vi "_Remote Set RF EN.vi"(4 "error in":errorcluster, 5 "RF EN (F)":bool, 6 "Q3? (F)":bool, 7 "Running (F)":bool) -> (0 "error out":errorcluster)   [LabVIEW 2012]
uses:
  Type/_RT Parameter.ctl
  Type/_RT Active Ch.ctl
  Type/_RT Expt.ctl
  Type/_Run Mode.ctl
  Type/_RT Mass Range.ctl
  Type/_RT Res Type.ctl
  Type/_RT Command.ctl
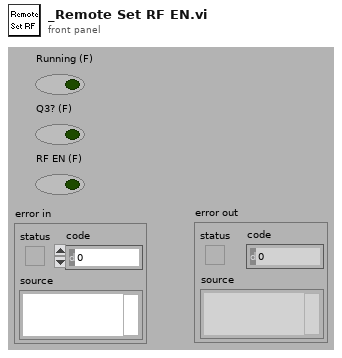
[diagram p1: front panel]
types:
  T1 = typedef "_RT Active Ch.ctl" = cluster{"Start":i32, "Step":i32, "ChID":i32}
  T2 = typedef "_RT Expt.ctl" = cluster{"StartT(mS)":i32, "#Cycles":i32, "Scan Type":T3, "PauseT(uS)":i32, "Polarity":u8, "DelayT(mS)":i32, "Active Ch":T1[], "Mass Range":T4[]}
  T3 = typedef "_Run Mode.ctl" = enum16{"MRM (Q1/Q2)", "Q1 Scan", "Q1 SRM", "Q2 Scan", "Q2 SRM", "Product Scan", "Precursor Scan", "Neutral Loss", "Neutral Gain"}
  T4 = typedef "_RT Mass Range.ctl" = cluster{"Steps":i32, "Dwell(uS)":i32, "Resolution Type":T5, "Ramping Ch":T1[]}
  T5 = typedef "_RT Res Type.ctl" = u16
  T6 = typedef "_RT Parameter.ctl" = cluster{"RunMode":i32, "Initial Ch":T1[], "Sync":u8, "Expt":T2[], "EqTime(mS)":i32}
  T7 = typedef "_RT Command.ctl" = enum16{"Start", "Stop", "Runtime Update", "Get Data", "Get Info", "Get Status", "Get Param", "Get Config", "Get Table", "Read ADC", "Set Oscillator", "Update Config", "Update Table", "Set All Pol", "Set Pol and DC", "Set Max Mass", "Toggle RP", "Toggle EL", "Set PIC", "Initialize Turbo", "Send Turbo Comm", "Close Turbo", "P1", "P2", "P3", "Send Serial", "Set LC Out", "Get LC In", "Read VAC", "Test Table", "Toggle Power", "Get Startup", "Set Startup", "Get ADC Table", "Set ADC Table", "Get Brief Status", "Get Detail Status", "Auxiliary Update", "Set CC Logics", "Set CC Input Logics"}
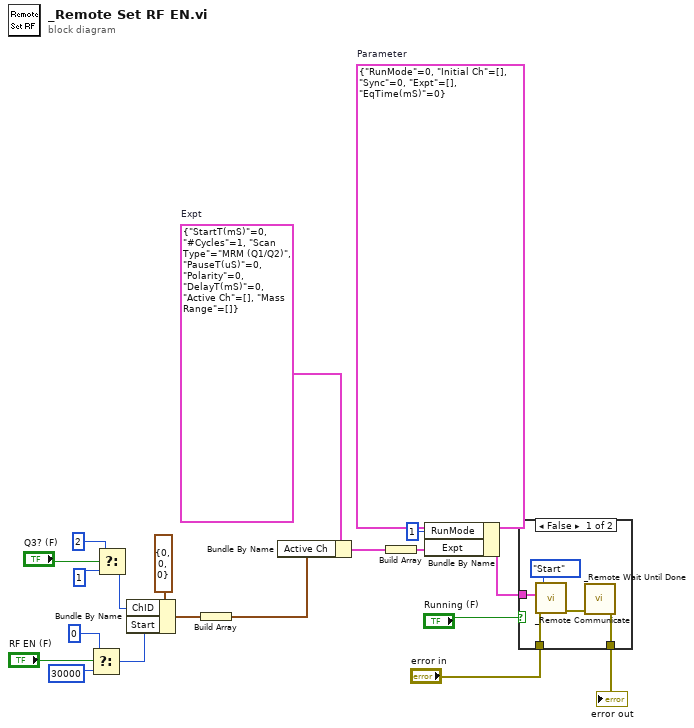
[diagram p0: block diagram]
diagram:
  w15 = T2 {"StartT(mS)"=0, "#Cycles"=1, "Scan Type"=enum."MRM (Q1/Q2)", "PauseT(uS)"=0, "Polarity"=0, "DelayT(mS)"=0, "Active Ch"=[], "Mass Range"=[]}  # Expt
  w18 = T6 {"RunMode"=0, "Initial Ch"=[], "Sync"=0, "Expt"=[], "EqTime(mS)"=0}  # Parameter
  n1 = Select(t=0 ("Start"), s="RF EN (F)", f=30000) -> (s? t:f=w3:i32)
  n2 = Select(t=2 ("ChID"), s="Q3? (F)", f=1 ("ChID")) -> (s? t:f=w7:i32)
  n3 = Bundle By Name(cluster=T1 {"Start"=0, "Step"=0, "ChID"=0} ("Active Channel"), "ChID"=w7, "Start"=w3) -> (w19:T1)
  n4 = Build Array(w19) -> (w6:T1[])
  n5 = Bundle By Name(cluster=w15, "Active Ch"=w6) -> (w14:T2)
  n6 = Build Array(w14) -> (w13:T2[])
  n7 = Bundle By Name(cluster=w18, "RunMode"=1, "Expt"=w13) -> (w17:T6)
  n8 = case shown="False" "Running (F)" {
    tunnel: [w25 w26] -> w20
    tunnel: w17 -> [w22 _]
    tunnel: "error in" -> [w21 w26]
    frame False {
      n9 = call "_Remote Communicate.vi"("error in (no error)"=w21, "Parameter"=w22, "Command"=_RT_Command."Start") -> ("error out"=w23:errorcluster)  [unwired: 3 in, 3 out]
      n10 = call "_Remote Wait Until Done.vi"("error IO"=w23) -> ("error out"=w25:errorcluster)  [unwired: 1 in, 1 out]
    }
    frame True {
    }
  }
  "error out" <- w20
